vi "test_Add Two Analog Inputs_FPGA Desktop Execution Node.vi"(8 "Error In":errorcluster, 9 "Count(Ticks)":u32, 10 "AI1":fxp<+/-,24,5>, 11 "AI0":fxp<+/-,24,5>) -> (0 "Error Out":errorcluster, 2 "AO0":fxp<+/-,20,5>)   [LabVIEW 2018]
uses:
  <vilib>/rvi/DesktopExecutionNode/Execution/niFpgaDEN_Execute.vi
  <vilib>/rvi/DesktopExecutionNode/DesktopExecutionNode.xnode
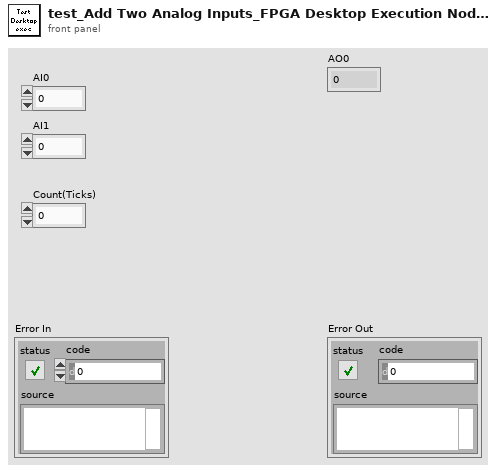
[diagram p1: front panel]
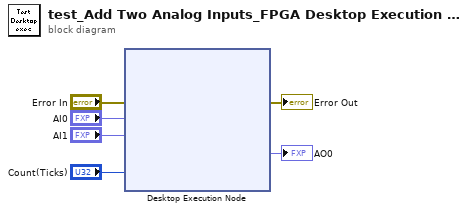
[diagram p0: block diagram]
diagram:
  n1 = xnode "Desktop Execution Node"("Error In"="Error In", "AI0"="AI0", "AI1"="AI1", "Count(Ticks)"="Count(Ticks)") -> ("Error Out"=→"Error Out":errorcluster, "AO0"=→"AO0":fxp<+/-,20,5>)
